vi "latlong_from-log.vi"(11 "log path":path) -> (1 "heading graph":dbl[](graph), 2 "Lat-Long":cluster{"X":dbl, "Y":dbl}[](graph), 3 "TM graph":cluster{"X":dbl, "Y":dbl}[](graph))   [LabVIEW 2019]
panel:
  out "x = y?":bool
  out "x-y":u32
  out "heading":dbl
  out "str2":string
  out "str1":string
  out "tm arr n":i32
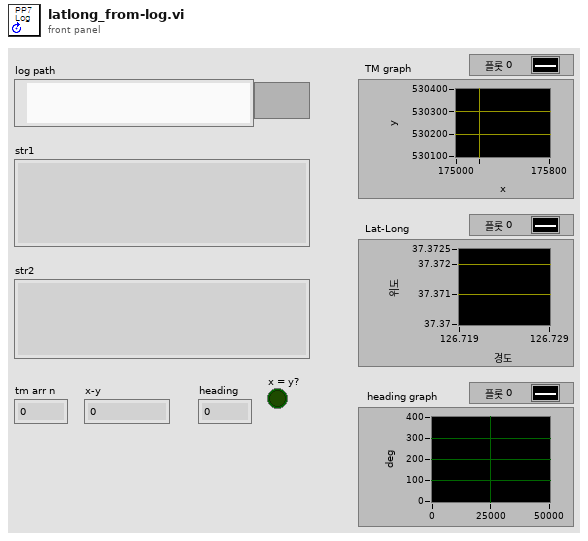
[diagram p1: front panel]
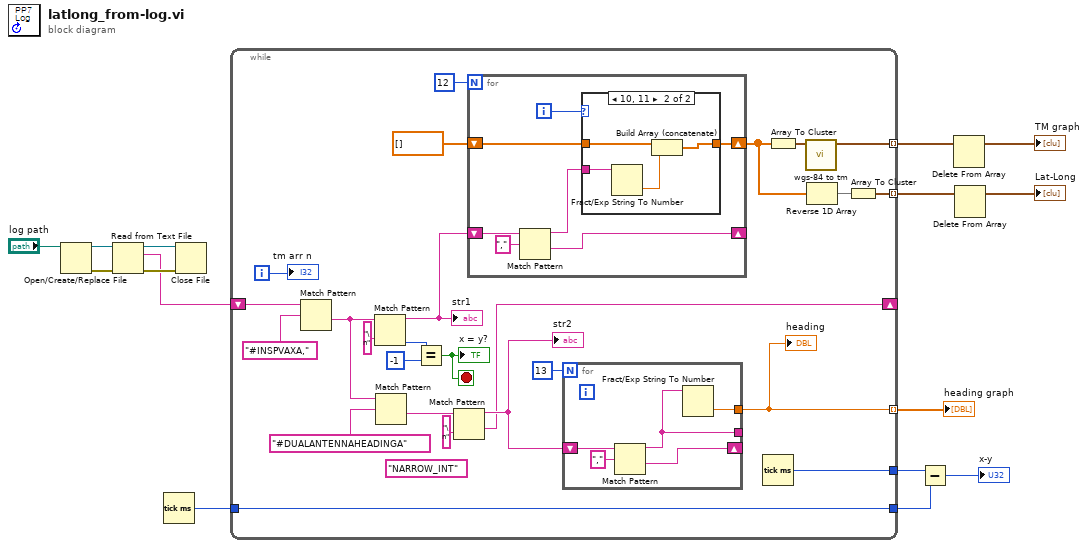
[diagram p0: block diagram]
diagram:
  n1 = Open/Create/Replace File(file path (use dialog)="log path") -> (refnum out=w14:refnum<file>, error out=w12:errorcluster)  [unwired: 5 in, 1 out]
  n2 = Read from Text File(file (use dialog)=w14, error in=w12) -> (refnum out=w13:refnum<file>, text=w10:string, error out=w11:errorcluster)  [unwired: 2 in, 1 out]
  n3 = Tick Count (ms)() -> (millisecond timer value=w8:u32)
  n4 = Close File(refnum=w13, error in=w11) -> ()  [unwired: 2 out]
  n5 = while {
    shift-right: [w26] -> _
    shift-left: w10 -> [w40]
    tunnel: [w25] -> w9 mode=indexing
    tunnel: [w21] -> w3 mode=indexing
    tunnel: [w22] -> w7
    tunnel: w8 -> [w22]
    tunnel: [w19] -> w6
    tunnel: [w16] -> w1 mode=indexing
    i -> [w17]
    stop <- w18 stop-if-true
    (unwired) "NARROW_INT" ("정규식")
    n6 = Match Pattern(string=w40, regular expression="#INSPVAXA," ("정규식")) -> (after substring=w34:string)  [unwired: 1 in, 3 out]
    n7 = Match Pattern(string=w34, regular expression="\n" ("정규식")) -> (before substring=w31:string, offset past match=w39:i32)  [unwired: 1 in, 2 out]
    "str1" <- w31
    n8 = Match Pattern(string=w34, regular expression="#DUALANTENNAHEADINGA" ("정규식")) -> (after substring=w32:string)  [unwired: 1 in, 3 out]
    n9 = Equal?(x=w39, y=-1) -> (x = y?=w18:bool)
    "x = y?" <- w18
    n10 = Match Pattern(string=w32, regular expression="\n" ("정규식")) -> (before substring=w27:string, after substring=w26:string)  [unwired: 1 in, 2 out]
    "str2" <- w27
    n11 = for {
      N: 12 ("숫자형") -> [_]
      shift-right: [w50] -> _
      shift-left: w31 -> [w52]
      shift-right: [w47] -> w23
      shift-left: dbl[] [] -> [w48]
      i -> [w49]
      n12 = Match Pattern(string=w52, regular expression="," ("정규식")) -> (before substring=w46:string, after substring=w50:string)  [unwired: 1 in, 2 out]
      n13 = case shown="10, 11" w49 {
        tunnel: w48 -> [w53 w57]
        tunnel: [w53 w56] -> w47
        tunnel: w46 -> [_ w55]
        frame 0, Default {
        }
        frame 10, 11 {
          n14 = Fract/Exp String To Number(string=w55) -> (number=w54:dbl)  [unwired: 3 in, 1 out]
          n15 = Build Array (concatenate)(w57, w54) -> (w56:dbl[])
        }
      }
    }
    n16 = for {
      N: 13 ("숫자형") -> [_]
      shift-right: [w43] -> _
      shift-left: w27 -> [w45]
      tunnel: [w42] -> _
      tunnel: [w41] -> w16
      n17 = Match Pattern(string=w45, regular expression="," ("정규식")) -> (before substring=w42:string, after substring=w43:string)  [unwired: 1 in, 2 out]
      n18 = Fract/Exp String To Number(string=w42) -> (number=w41:dbl)  [unwired: 3 in, 1 out]
    }
    "heading" <- w16
    n19 = Tick Count (ms)() -> (millisecond timer value=w19:u32)
    n20 = Array To Cluster(array=w23) -> (cluster=w24:cluster{"[0]":dbl, "[1]":dbl})
    n21 = call "wgs-84 to tm.vi"("in_lon-lat"=w24) -> ("TM"=w25:cluster{"Y(E)":dbl, "X(N)":dbl})  [unwired: 10 in]
    n22 = Reverse 1D Array(array=w23) -> (reversed array=w20:dbl[])
    n23 = Array To Cluster(array=w20) -> (cluster=w21:cluster{"[0]":dbl, "[1]":dbl})
    "tm arr n" <- w17
  }
  "heading graph" <- w1
  n24 = Subtract(x=w6, y=w7) -> (x-y=→"x-y":u32)
  n25 = Delete From Array(array=w9) -> (array with subset deleted=→"TM graph":cluster{"Y(E)":dbl, "X(N)":dbl}[])  [unwired: 2 in, 1 out]
  n26 = Delete From Array(array=w3) -> (array with subset deleted=→"Lat-Long":cluster{"[0]":dbl, "[1]":dbl}[])  [unwired: 2 in, 1 out]
